vi "setUp.vi"(8 "error in (no error)":errorcluster, 11 "reference in":refnum<class "Test TCP Nested Endpoint Nonforwarded Messages.lvclass">) -> (0 "error out":errorcluster, 3 "reference out":refnum<class "Test TCP Nested Endpoint Nonforwarded Messages.lvclass">)   [LabVIEW 2020, in "Test TCP Nested Endpoint Nonforwarded Messages.lvclass"]
doc: "setUp runs prior to the test method during test execution. Use this method to initialize any object data required by your tests."
uses:
  Test TCP Nested Endpoint Nonforwarded Messages.lvclass
  <vilib>/addons/_JKI Toolkits/VI Tester/TestCase.llb/TestCase.lvclass
  <vilib>/ActorFramework/Actor/Actor.lvclass
  <vilib>/ActorFramework/Message Queue/Message Queue.lvclass
  Source/Protocols/TCP Strategy/TCP Stream Initiator/TCP Stream Initiator.lvclass
  Source/Protocols/TCP Strategy/TCP Stream/TCP Stream.lvclass
  Source/Ciphers/AES/AES.lvclass
  Source/Ciphers/AES/Ton Plomp Encryption/AES-Modes.ctl
  Source/Ciphers/AES/Ton Plomp Encryption/Encryption.lvlib
  Source/Protocols/TCP Strategy/TCP Stream Listener/TCP Stream Listener.lvclass
  Source/Nested Endpoint/Nested Endpoint/Nested Endpoint.lvclass
  Source/Network Endpoint/Network Endpoint/Network Endpoint.lvclass
  Source/Abstract Classes/Message Stream/Message Stream.lvclass
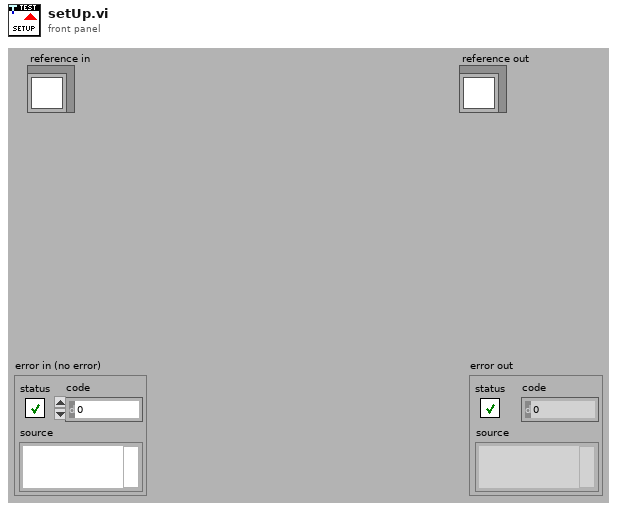
[diagram p1: front panel]
types:
  T1 = typedef "Encryption.lvlib/AES-Modes.ctl" = enum16{"ECB", "CBC", "CFB128", "OFB"}
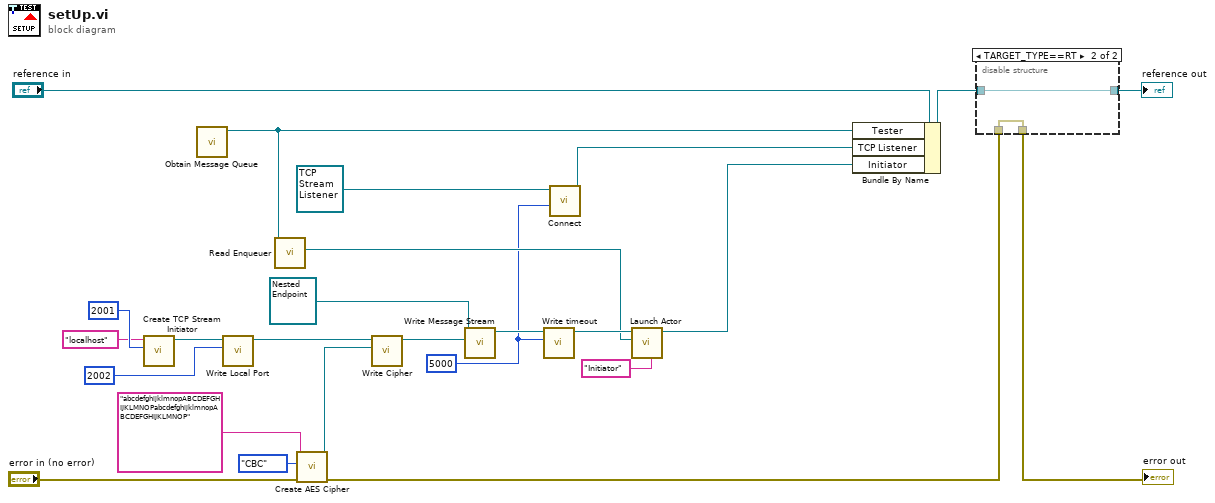
[diagram p0: block diagram]
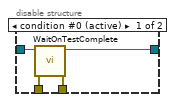
[diagram p2: hidden frame]
diagram:
  w2 = 5000 ("timeout")
  n1 = call "Create TCP Stream Initiator.vi"("Remote Port"=u16 2001 ("Port"), "Remote Address"="localhost" ("IP Address")) -> ("TCP Stream Initiator"=w21:refnum<class "TCP Stream Initiator.lvclass">)  [unwired: 9 in]
  n2 = call <vilib>:"Obtain Message Queue.vi"() -> ("Message Queue"=w10:refnum<class "Message Queue.lvclass">)  [unwired: 10 in, 1 out]
  n3 = call "Write Local Port.vi"("local port"=u16 2002, "TCP Stream in"=w21) -> ("TCP Stream out"=w19:refnum<class "TCP Stream Initiator.lvclass">)  [unwired: 9 in]
  n4 = call <vilib>:"Read Enqueuer.vi"("Message Queue"=w10) -> ("Message Enqueuer"=w5:refnum<class "Message Enqueuer.lvclass">)  [unwired: 10 in]
  n5 = call "Create AES Cipher.vi"("error in (no error)"="error in (no error)", "Operation Mode"=AES-Modes."CBC", "Cipher Key"="abcdefghijklmnopABCDEFGHIJKLMNOPabcdefghijklmnopABCDEFGHIJKLMNOP") -> ("error out"=w15:errorcluster, "AES out"=w14:refnum<class "AES.lvclass">)  [unwired: 7 in]
  n6 = call "Write Cipher.vi"("Cipher"=w14, "Message Stream in"=w19) -> ("Message Stream out"=w13:refnum<class "TCP Stream Initiator.lvclass">)  [unwired: 9 in]
  n7 = call "Write Message Stream.vi"("Message Stream"=w13, "Network Endpoint in"=refnum<class "Nested Endpoint.lvclass"> refnum ("Nested Endpoint.lvlib:Nested Endpoint.lvclass")) -> ("Network Endpoint out"=w8:refnum<class "Nested Endpoint.lvclass">)  [unwired: 9 in]
  n8 = call "Write timeout.vi"("timeout"=w2, "Network Endpoint in"=w8) -> ("Network Endpoint out"=w7:refnum<class "Nested Endpoint.lvclass">)  [unwired: 9 in]
  n9 = call-dynamic "Connect.vi"("timeout"=w2, "TCP Stream Listener in"=refnum<class "TCP Stream Listener.lvclass"> refnum ("TCP Stream Listener.lvclass")) -> ("TCP Stream Listener out"=w1:refnum<class "TCP Stream Listener.lvclass">)  [unwired: 8 in, 1 out]
  n10 = call <vilib>:"Launch Actor.vi"("Debug Alias"="Initiator", "Actor-to-Caller Enqueuer"=w5, "Actor"=w7) -> ("Caller-To-Actor Enqueuer"=w11:refnum<class "Message Enqueuer.lvclass">)  [unwired: 7 in, 1 out]
  n11 = Bundle By Name(cluster="reference in", "Tester"=w10, "TCP Listener"=w1, "Initiator"=w11) -> (w22:refnum<class "Test TCP Nested Endpoint Nonforwarded Messages.lvclass">)
  n12 = disable-structure shown="TARGET_TYPE==RT" {
    disable-tunnel: w15 -> [w29 w30]
    disable-tunnel: [w28 w30] -> w25
    disable-tunnel: [w27 w31] -> w23
    disable-tunnel: w22 -> [w26 w31]
    frame condition #0 (active) {
      n13 = call <vilib>:"WaitOnTestComplete.vi"("error in (no error)"=w29, "TestCase in"=w26) -> ("error out"=w28:errorcluster, "TestCase out"=w27:refnum<class "Test TCP Nested Endpoint Nonforwarded Messages.lvclass">)  [unwired: 8 in]
    }
    frame condition #1 {
    }
  }
  "error out" <- w25
  "reference out" <- w23
